vi "test_python.vi"() -> ()   [LabVIEW 2020]
panel:
  out "Super Res":dbl[][](graph)
  out "Low Res":dbl[][](graph)
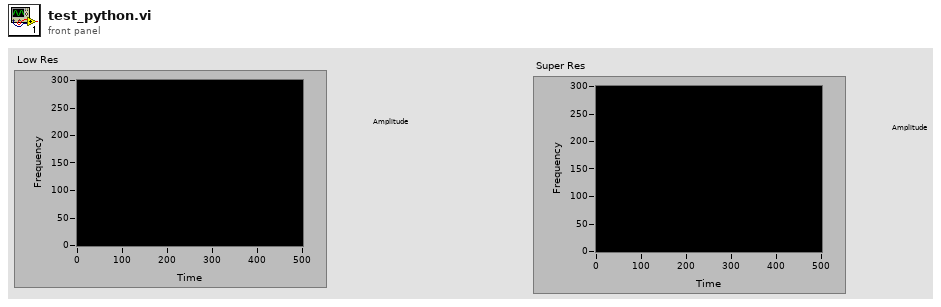
[diagram p1: front panel]
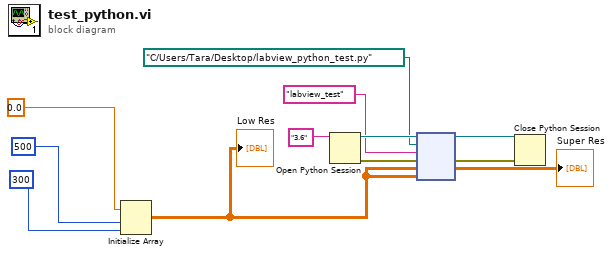
[diagram p0: block diagram]
diagram:
  n1 = Initialize Array(0.0, 500, 300) -> (w5:dbl[][])
  "Low Res" <- w5
  n2 = Open Python Session(python version="3.6") -> (session out=w9:refnum<k35>, error out=w7:errorcluster)  [unwired: 2 in]
  n3 = node(w9, path "C:/Users/Tara/Desktop/labview_python_test.py", "labview_test", w7, w5, w5) -> (w8:refnum<k35>, w6:errorcluster, →"Super Res":dbl[][])  [unwired: 1 in, 2 out]
  n4 = Close Python Session(session in=w8, error in=w6) -> ()  [unwired: 1 out]
